vi "Select All Write.vi"(4 "error in (no error)":errorcluster, 5 "Value":enum16{"Check All", "Uncheck All"}(ring), 6 "Container State":T2, 7 "Display State In":T1) -> (0 "error out":errorcluster, 3 "Display State Out":T1)   [LabVIEW 2018, in "ListBox XControl.xctl"]
uses:
  ListBox XControl.xctl
  <vilib>/_xctls/Container State.ctl
  State ListBox.ctl
  <vilib>/_xctls/XControlSupport.lvlib
panel:
  in  "Enum":enum16{"Check All", "Uncheck All"}(ring)
  # "Replace the Value Control below with a Control of desired type.\nDo not remove this Control or the others from the connector pane.\nDo not change the connector pane pattern.\nThe Value control should always be the third terminal from top on the input side in the connector pane."
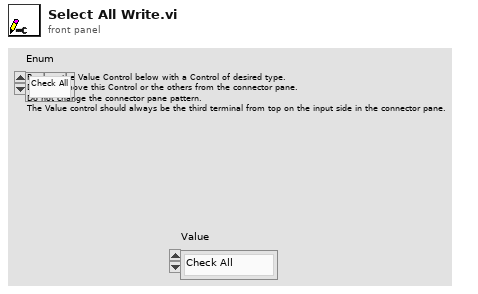
[diagram p1: front panel]
types:
  T1 = typedef "ListBox XControl.xctl/State ListBox.ctl" = cluster{"ItemNames[]":string[], "Listbox Ref":refnum<vi>, "Select All By Default":bool}
  T2 = typedef "XControlSupport.lvlib/Container State.ctl" = cluster{"Indicator?":bool, "Run Mode?":bool, " Refnum":refnum<vi>}
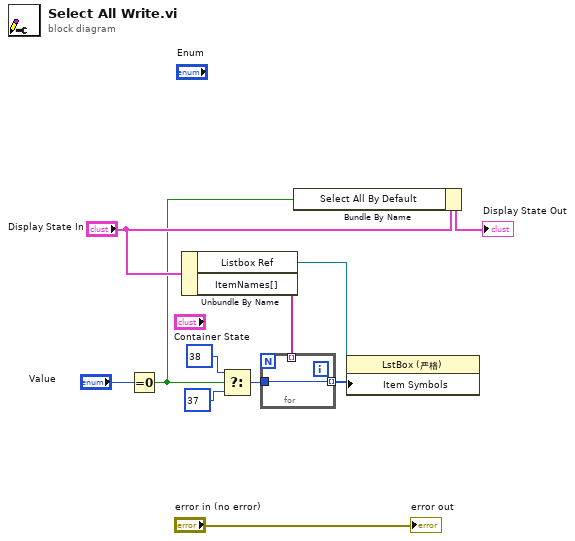
[diagram p0: block diagram]
diagram:
  n1 = Equal To 0?(x="Value") -> (x = 0?=w1:bool)
  n2 = Unbundle By Name("Display State In") -> ("Listbox Ref"=w10:refnum<vi>, "ItemNames[]"=w9:string[])
  n3 = Select(t=38, s=w1, f=37) -> (s? t:f=w5:i32)
  n4 = for {
    tunnel: w9 -> [_] mode=indexing
    tunnel: [w12] -> w8 mode=indexing
    tunnel: w5 -> [w12]
  }
  n5 = Bundle By Name(cluster="Display State In", "Select All By Default"=w1) -> (→"Display State Out":T1)
  n6 = property class="LstBox (严格)"(reference=w10, "Item Symbols"=w8) -> ()  [unwired: 1 in, 2 out]
  "error out" <- "error in (no error)"
